vi "Panther Dashboard--global.vi"() -> ()   [LabVIEW 2019, in "Panther Dashboard.lvlib"]
uses:
  Panther Dashboard.lvlib
panel:
  in  "Target":string
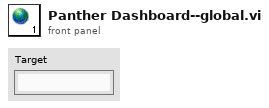
[diagram p1: front panel]
diagram:
